vi "Parse Request-JSONtext.vi"(8 "error in (no error)":errorcluster, 10 "{JSON} Request":string) -> (0 "error out":errorcluster, 1 "params":string, 2 "method":string, 4 "id":string)   [LabVIEW 2019, in "JSON-RPC.lvclass"]
uses:
  JSON-RPC.lvclass
  523bbeac-5bfa-4355-a479-ec0e355c2dae.vi
  5dfc14ef-dff6-4e36-b5f1-09fb62becacc.vi
  f339b867-7010-45a6-b71e-b2a9da4366e1.vi
  <vilib>/JDP Science/JSONtext/Find Item.vi
  <vilib>/JDP Science/JSONtext/String Subset.vi
  <vilib>/JDP Science/JSONtext/Parsing/Parse Full Path or Item Name.vi
  <vilib>/JDP Science/JSONtext/Next JSON Value.vi
  <vilib>/JDP Science/JSONtext/support/Error Cluster From Code.vi
  <vilib>/JDP Science/JSONtext/Offset/Find Item Locations by Path.vi
  <vilib>/JDP Science/JSONtext/JSON text to Variant.vi
  <vilib>/JDP Science/JSONtext/LVClass Serializer/JSONtext LVClass Serializer.lvclass
  <vilib>/JDP Science/JSONtext/JSONtext.lvlib
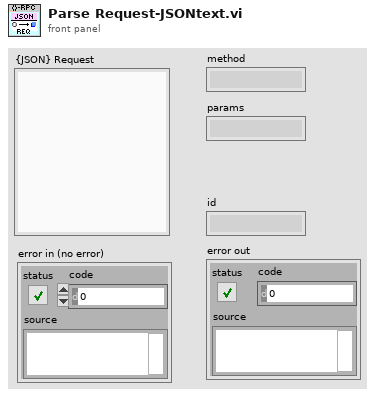
[diagram p1: front panel]
types:
  T1 = cluster{"jsconrpc":string, "method":string, "params":string, "id":string}
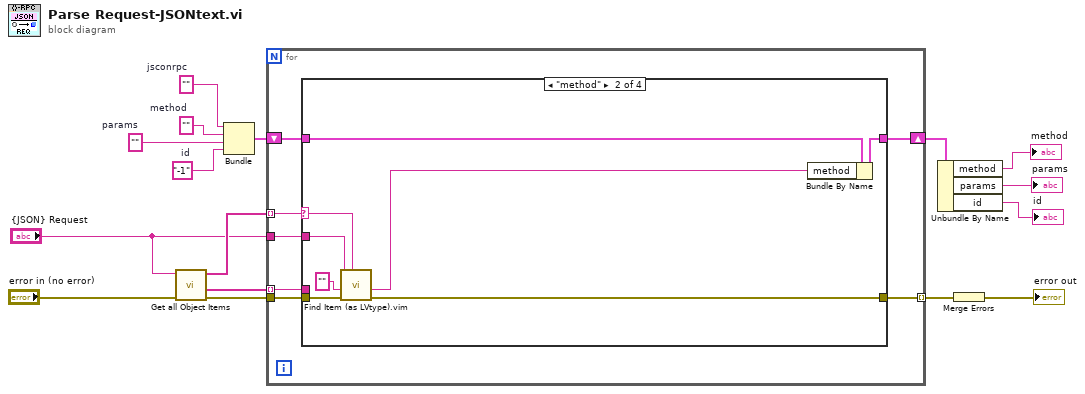
[diagram p0: block diagram]
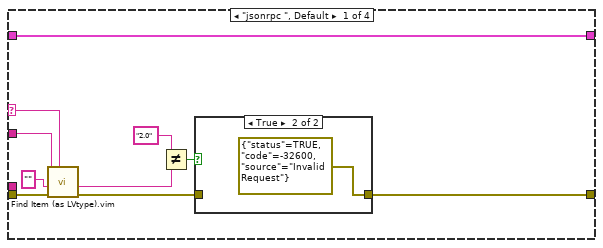
[diagram p2: hidden frame]
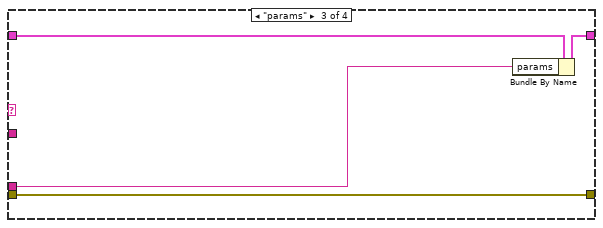
[diagram p4: hidden frame]
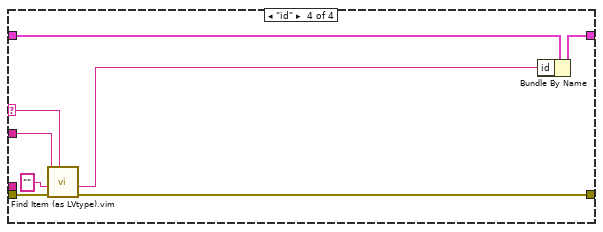
[diagram p5: hidden frame]
diagram:
  w14 = "-1"  # id
  w13 = ""  # params
  w12 = ""  # jsconrpc
  w11 = ""  # method
  n1 = call <vilib>:"Get all Object Items.vi"("error in (no error)"="error in (no error)", "JSON"="{JSON} Request") -> ("error out"=w8:errorcluster, "<JSON>"=w3:string[], "Item Names"=w10:string[])  [unwired: 6 in, 1 out]
  n2 = Bundle("jsconrpc"=w12, "method"=w11, "params"=w13, "id"=w14) -> (w15:T1)  [unwired: 1 in]
  n3 = for {
    tunnel: w3 -> [w22] mode=indexing
    tunnel: w10 -> [w23] mode=indexing
    tunnel: w8 -> [w21]
    tunnel: [w20] -> w9 mode=indexing
    tunnel: "{JSON} Request" -> [w19]
    shift-right: [w17] -> w16
    shift-left: w15 -> [w18]
    n4 = case shown="\"method\"" w23 {
      selector: w23 -> [w28 w41 _ w55]
      tunnel: w22 -> [_ _ w44 _]
      tunnel: w21 -> [w30 w43 w45 w54]
      tunnel: [w31 w40 w45 w53] -> w20
      tunnel: w19 -> [w24 w36 _ w48]
      tunnel: w18 -> [w25 w39 w47 w51]
      tunnel: [w25 w38 w46 w50] -> w17
      frame "jsonrpc ", Default {
        n5 = call "Find Item (as LVtype).vim"("$Path or Item Name"=w28, "error in (no error)"=w30, "Data Type and Default Value"="" ("x"), "JSON"=w24) -> ("error out"=w29:errorcluster, "Data"=w27:string)  [unwired: 4 in, 2 out]
        n6 = Not Equal?(x="2.0", y=w27) -> (x != y?=w32:bool)
        n7 = case shown="True" w32 {
          tunnel: w29 -> [w34 _]
          tunnel: [w34 errorcluster {"status"=TRUE, "code"=-32600, "source"="Invalid Request"} ("error out")] -> w31
          frame False {
          }
          frame True {
          }
        }
      }
      frame "method" {
        n8 = call "Find Item (as LVtype).vim"("$Path or Item Name"=w41, "error in (no error)"=w43, "Data Type and Default Value"="" ("x"), "JSON"=w36) -> ("error out"=w40:errorcluster, "Data"=w37:string)  [unwired: 4 in, 2 out]
        n9 = Bundle By Name(cluster=w39, "method"=w37) -> (w38:T1)
      }
      frame "params" {
        n10 = Bundle By Name(cluster=w47, "params"=w44) -> (w46:T1)
      }
      frame "id" {
        n11 = call "Find Item (as LVtype).vim"("$Path or Item Name"=w55, "error in (no error)"=w54, "Data Type and Default Value"="", "JSON"=w48) -> ("error out"=w53:errorcluster, "Data"=w49:string)  [unwired: 4 in, 2 out]
        n12 = Bundle By Name(cluster=w51, "id"=w49) -> (w50:T1)
      }
    }
  }
  n13 = Unbundle By Name(w16) -> ("method"=→"method":string, "params"=→"params":string, "id"=→"id":string)
  n14 = Merge Errors(w9) -> (→"error out":errorcluster)
